vi "Init.vi"(8 "error in (no error)":errorcluster, 10 "Measurement":string) -> (0 "error out":errorcluster, 3 "DataPoint out":refnum<class "DataPoint.lvclass">)   [LabVIEW 2018, in "InfluxDB Client.lvlib" / "DataPoint.lvclass"]
uses:
  DataPoint.lvclass
  Controls/Precision.ctl
  Controls/TagSet.ctl
  Controls/FieldSet.ctl
  DataPoint.lvclass/DataPoint.ctl
  InfluxDB Client.lvlib
panel:
  in  "DataPoint in":refnum<class "DataPoint.lvclass">
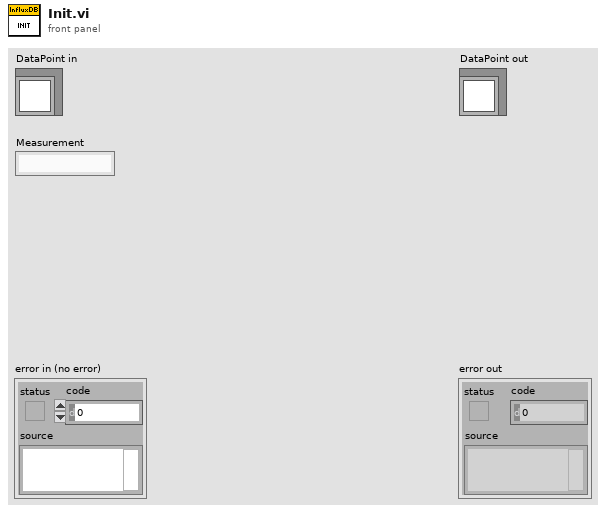
[diagram p1: front panel]
types:
  T1 = typedef "InfluxDB Client.lvlib/FieldSet.ctl" = cluster{"Key":string, "Value":variant}
  T2 = typedef "InfluxDB Client.lvlib/TagSet.ctl" = cluster{"Key":string, "Value":string}
  T3 = typedef "InfluxDB Client.lvlib/Precision.ctl" = enum16{"Seconds", "Milliseconds", "Nanoseconds"}
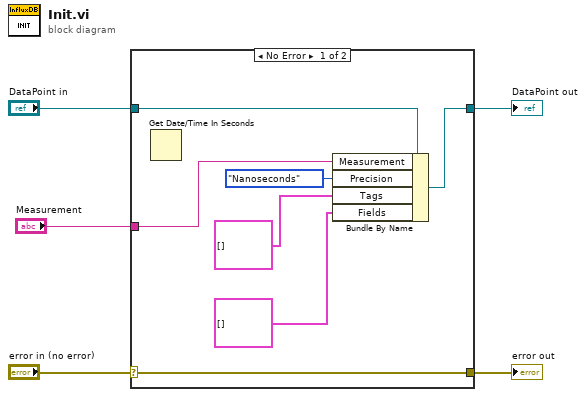
[diagram p0: block diagram]
diagram:
  n1 = case shown="No Error" "error in (no error)" {
    selector: "error in (no error)" -> [w12 w14]
    tunnel: [w12 w14] -> w4
    tunnel: "DataPoint in" -> [w11 w13]
    tunnel: [w10 w13] -> w2
    tunnel: "Measurement" -> [w9 _]
    frame No Error {
      n2 = Get Date/Time In Seconds() -> ()  [unwired: 1 out]
      n3 = Bundle By Name(cluster=w11, "Measurement"=w9, "Precision"=Precision."Nanoseconds", "Tags"=T2[] [], "Fields"=T1[] []) -> (w10:refnum<class "DataPoint.lvclass">)
    }
    frame Error {
    }
  }
  "error out" <- w4
  "DataPoint out" <- w2
